vi "Blank VI 04.vi"(7 "Calling VI Ref":refnum<vi>) -> ()   [LabVIEW 2016]
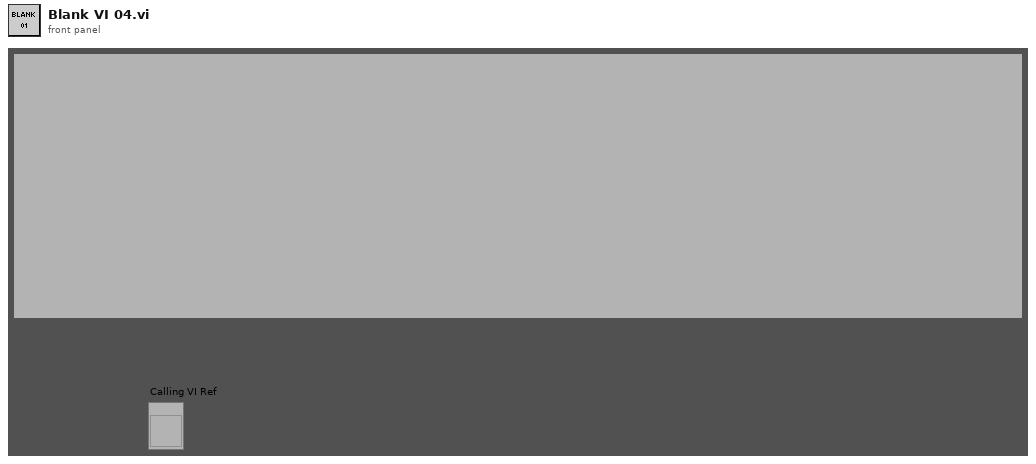
[diagram p1: front panel]
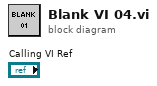
[diagram p0: block diagram]
diagram:
